vi "Create All Message Queues.vi"(8 "error in (no error)":errorcluster) -> (0 "error out":errorcluster, 3 "Message Queues Out":T1)   [LabVIEW 2014, in "WINFAS 2 Message Queue.lvlib"]
doc: "This VI creates and initializes all the message queues for your application. If your application requires more than one message queue, right-click the \"Message Queues\" constant above and select Open Type Def. Add the new Message Queue(s) to the type definition, then initialize them in this VI."
uses:
  WINFAS 2 Message Queue.lvlib
  All Message Queues.ctl
  Message Cluster.ctl
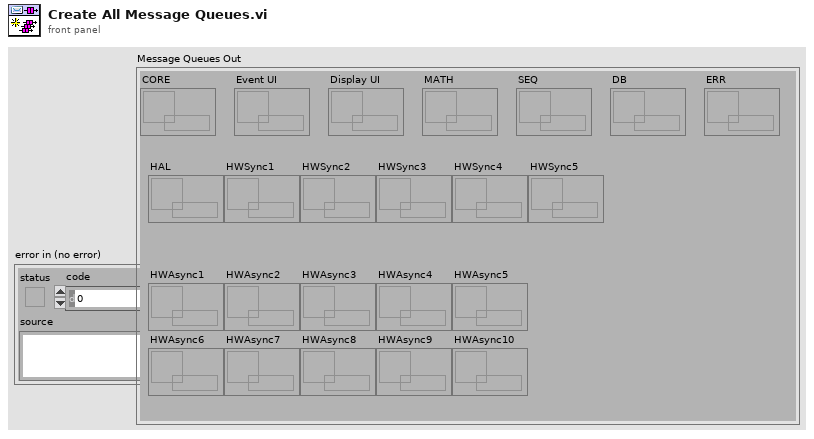
[diagram p1: front panel]
types:
  T1 = typedef "WINFAS 2 Message Queue.lvlib/All Message Queues.ctl" = cluster{"CORE":refnum<queue>, "Event UI":refnum<queue>, "Display UI":refnum<queue>, "MATH":refnum<queue>, "SEQ":refnum<queue>, "DB":refnum<queue>, "ERR":refnum<queue>, "HAL":refnum<queue>, "HWSync1":refnum<queue>, "HWSync2":refnum<queue>, "HWSync3":refnum<queue>, "HWSync4":refnum<queue>, "HWSync5":refnum<queue>, "HWAsync1":refnum<queue>, "HWAsync2":refnum<queue>, "HWAsync3":refnum<queue>, "HWAsync4":refnum<queue>, "HWAsync5":refnum<queue>, "HWAsync6":refnum<queue>, "HWAsync7":refnum<queue>, "HWAsync8":refnum<queue>, "HWAsync9":refnum<queue>, "HWAsync10":refnum<queue>}
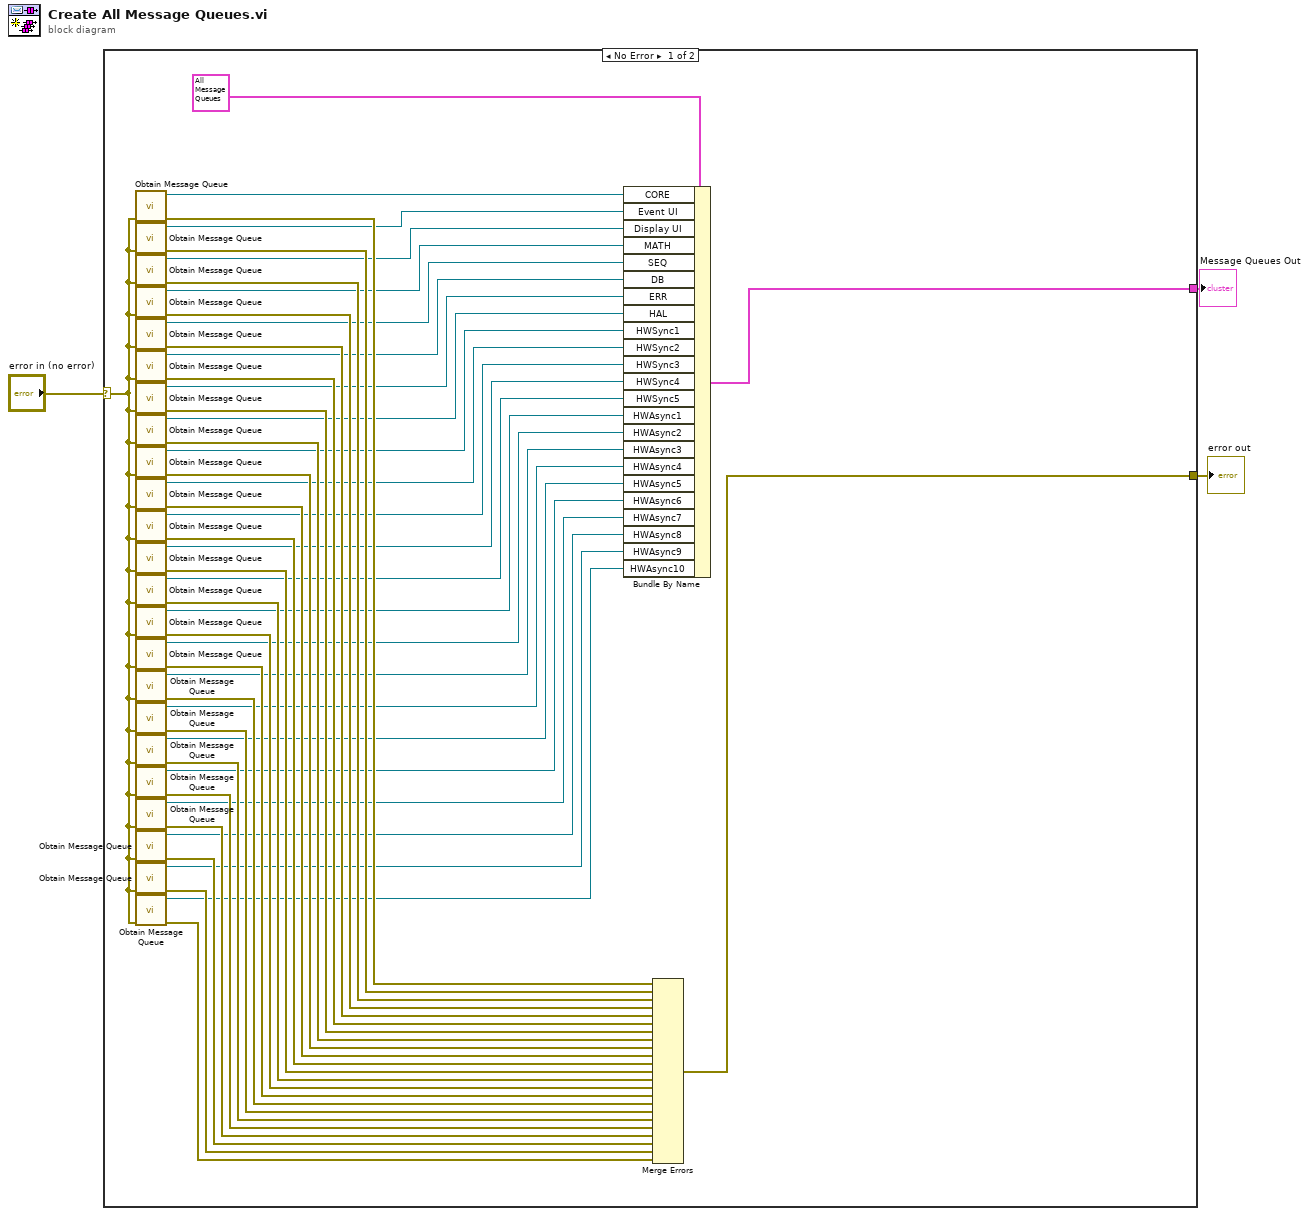
[diagram p0: block diagram]
diagram:
  n1 = case shown="No Error" "error in (no error)" {
    selector: "error in (no error)" -> [w24 w54]
    tunnel: [w39 w54] -> w3
    tunnel: [w40 _] -> w1
    frame No Error {
      n2 = call "Obtain Message Queue.vi"("error in (no error)"=w24) -> ("error out"=w53:errorcluster, "Message Queue"=w38:refnum<queue>)  [unwired: 9 in]
      n3 = call "Obtain Message Queue.vi"("error in (no error)"=w24) -> ("error out"=w52:errorcluster, "Message Queue"=w37:refnum<queue>)  [unwired: 9 in]
      n4 = call "Obtain Message Queue.vi"("error in (no error)"=w24) -> ("error out"=w51:errorcluster, "Message Queue"=w36:refnum<queue>)  [unwired: 9 in]
      n5 = call "Obtain Message Queue.vi"("error in (no error)"=w24) -> ("error out"=w50:errorcluster, "Message Queue"=w35:refnum<queue>)  [unwired: 9 in]
      n6 = call "Obtain Message Queue.vi"("error in (no error)"=w24) -> ("error out"=w49:errorcluster, "Message Queue"=w34:refnum<queue>)  [unwired: 9 in]
      n7 = call "Obtain Message Queue.vi"("error in (no error)"=w24) -> ("error out"=w48:errorcluster, "Message Queue"=w33:refnum<queue>)  [unwired: 9 in]
      n8 = call "Obtain Message Queue.vi"("error in (no error)"=w24) -> ("error out"=w47:errorcluster, "Message Queue"=w32:refnum<queue>)  [unwired: 9 in]
      n9 = call "Obtain Message Queue.vi"("error in (no error)"=w24) -> ("error out"=w46:errorcluster, "Message Queue"=w31:refnum<queue>)  [unwired: 9 in]
      n10 = call "Obtain Message Queue.vi"("error in (no error)"=w24) -> ("error out"=w45:errorcluster, "Message Queue"=w30:refnum<queue>)  [unwired: 9 in]
      n11 = call "Obtain Message Queue.vi"("error in (no error)"=w24) -> ("error out"=w44:errorcluster, "Message Queue"=w29:refnum<queue>)  [unwired: 9 in]
      n12 = call "Obtain Message Queue.vi"("error in (no error)"=w24) -> ("error out"=w43:errorcluster, "Message Queue"=w28:refnum<queue>)  [unwired: 9 in]
      n13 = call "Obtain Message Queue.vi"("error in (no error)"=w24) -> ("error out"=w42:errorcluster, "Message Queue"=w27:refnum<queue>)  [unwired: 9 in]
      n14 = call "Obtain Message Queue.vi"("error in (no error)"=w24) -> ("error out"=w41:errorcluster, "Message Queue"=w25:refnum<queue>)  [unwired: 9 in]
      n15 = call "Obtain Message Queue.vi"("error in (no error)"=w24) -> ("error out"=w23:errorcluster, "Message Queue"=w13:refnum<queue>)  [unwired: 9 in]
      n16 = call "Obtain Message Queue.vi"("error in (no error)"=w24) -> ("error out"=w22:errorcluster, "Message Queue"=w12:refnum<queue>)  [unwired: 9 in]
      n17 = call "Obtain Message Queue.vi"("error in (no error)"=w24) -> ("error out"=w21:errorcluster, "Message Queue"=w11:refnum<queue>)  [unwired: 9 in]
      n18 = call "Obtain Message Queue.vi"("error in (no error)"=w24) -> ("error out"=w20:errorcluster, "Message Queue"=w10:refnum<queue>)  [unwired: 9 in]
      n19 = call "Obtain Message Queue.vi"("error in (no error)"=w24) -> ("error out"=w19:errorcluster, "Message Queue"=w9:refnum<queue>)  [unwired: 9 in]
      n20 = call "Obtain Message Queue.vi"("error in (no error)"=w24) -> ("error out"=w18:errorcluster, "Message Queue"=w8:refnum<queue>)  [unwired: 9 in]
      n21 = call "Obtain Message Queue.vi"("error in (no error)"=w24) -> ("error out"=w17:errorcluster, "Message Queue"=w7:refnum<queue>)  [unwired: 9 in]
      n22 = call "Obtain Message Queue.vi"("error in (no error)"=w24) -> ("error out"=w16:errorcluster, "Message Queue"=w6:refnum<queue>)  [unwired: 9 in]
      n23 = call "Obtain Message Queue.vi"("error in (no error)"=w24) -> ("error out"=w15:errorcluster, "Message Queue"=w5:refnum<queue>)  [unwired: 9 in]
      n24 = call "Obtain Message Queue.vi"("error in (no error)"=w24) -> ("error out"=w14:errorcluster, "Message Queue"=w4:refnum<queue>)  [unwired: 9 in]
      n25 = Bundle By Name(cluster=T1 {"CORE"=refnum, "Event UI"=refnum, "Display UI"=refnum, "MATH"=refnum, "SEQ"=refnum, "DB"=refnum, "ERR"=refnum, "HAL"=refnum, "HWSync1"=refnum, "HWSync2"=refnum, "HWSync3"=refnum, "HWSync4"=refnum, "HWSync5"=refnum, "HWAsync1"=refnum, "HWAsync2"=refnum, "HWAsync3"=refnum, "HWAsync4"=refnum, "HWAsync5"=refnum, "HWAsync6"=refnum, "HWAsync7"=refnum, "HWAsync8"=refnum, "HWAsync9"=refnum, "HWAsync10"=refnum} ("Message Queues"), "CORE"=w38, "Event UI"=w37, "Display UI"=w36, "MATH"=w35, "SEQ"=w34, "DB"=w33, "ERR"=w32, "HAL"=w31, "HWSync1"=w30, "HWSync2"=w29, "HWSync3"=w28, "HWSync4"=w27, "HWSync5"=w25, "HWAsync1"=w13, "HWAsync2"=w12, "HWAsync3"=w11, "HWAsync4"=w10, "HWAsync5"=w9, "HWAsync6"=w8, "HWAsync7"=w7, "HWAsync8"=w6, "HWAsync9"=w5, "HWAsync10"=w4) -> (w40:T1)
      n26 = Merge Errors(w53, w52, w51, w50, w49, w48, w47, w46, w45, w44, w43, w42, w41, w23, w22, w21, w20, w19, w18, w17, w16, w15, w14) -> (w39:errorcluster)
    }
    frame Error {
    }
  }
  "error out" <- w3
  "Message Queues Out" <- w1
